vi "Ticks to Dist.vi"(8 "error in (no error)":errorcluster, 10 "ticks":i32, 11 "KUKA youBot gripper motor_EtherCAT in":refnum<class "NI_Robotics_KUKA youBot Gripper Motor_EtherCAT.lvclass">) -> (0 "error out":errorcluster, 2 "distance (m)":dbl, 3 "KUKA youBot gripper motor_EtherCAT out":refnum<class "NI_Robotics_KUKA youBot Gripper Motor_EtherCAT.lvclass">)   [LabVIEW 2017, in "NI_Robotics_KUKA youBot Host.lvlib" / "NI_Robotics_KUKA youBot Gripper Motor_EtherCAT.lvclass"]
uses:
  <vilib>/robotics/KUKA youBot/Motor/Gripper Motor EtherCAT/NI_Robotics_KUKA youBot Gripper Motor_EtherCAT.lvclass
  <vilib>/robotics/KUKA youBot/Motor/Gripper Motor EtherCAT/NI_Robotics_KUKA youBot Gripper Motor_EtherCAT.lvclass/NI_Robotics_KUKA youBot Gripper Motor_EtherCAT.ctl
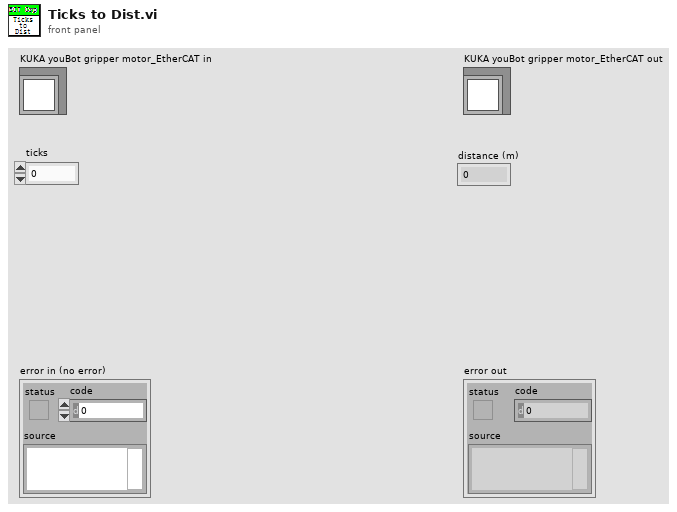
[diagram p1: front panel]
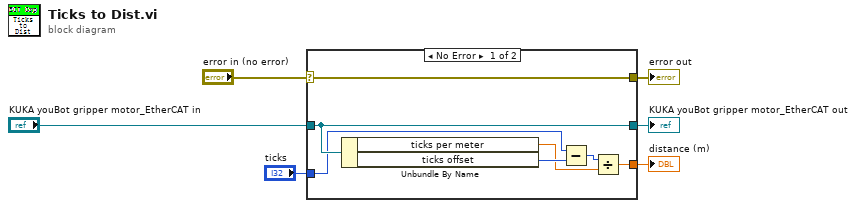
[diagram p0: block diagram]
diagram:
  n1 = case shown="No Error" "error in (no error)" {
    selector: "error in (no error)" -> [w13 w15]
    tunnel: [w13 w15] -> w5
    tunnel: [w12 w14] -> w3
    tunnel: "KUKA youBot gripper motor_EtherCAT in" -> [w12 w14]
    tunnel: "ticks" -> [w11 _]
    tunnel: [w7 _] -> w1
    frame No Error {
      n2 = Unbundle By Name(w12) -> ("ticks per meter"=w8:dbl, "ticks offset"=w10:i32)
      n3 = Subtract(x=w11, y=w10) -> (x-y=w9:i32)
      n4 = Divide(x=w9, y=w8) -> (x/y=w7:dbl)
    }
    frame Error {
    }
  }
  "error out" <- w5
  "KUKA youBot gripper motor_EtherCAT out" <- w3
  "distance (m)" <- w1
